vi "RT Driver VI.vi"(7 "Operation":T1, 11 "Device Reference in":T2 format="%.0x") -> (0 "Error Code":i32)   [LabVIEW 2017, in "Data Sharing Custom Device Engine.lvlib"]
uses:
  Data Sharing Custom Device Engine.lvlib
  <vilib>/NI Veristand/Custom Device API/Custom Device Item Ref.ctl
  <vilib>/NI Veristand/Custom Device API/Hardware Interface Driver VI Operation.ctl
  Builds/Data Sharing Framework/Current/Data Sharing Framework Core/Data Sharing Framework Core.lvlibp/Engine/Framework/Framework.lvclass
  Builds/Data Sharing Framework/Current/Data Sharing Framework Core/Data Sharing Framework Core.lvlibp/Engine/Internal/Configuration Classes/Framework Configuration/Framework Configuration.lvclass
  <vilib>/NI Veristand/Custom Device API/Custom Device API.lvlib
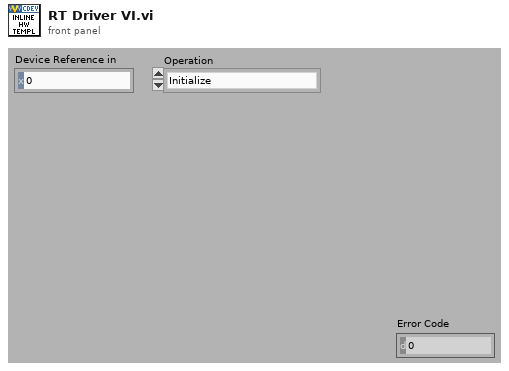
[diagram p1: front panel]
types:
  T1 = typedef "Custom Device API.lvlib/Hardware Interface Driver VI Operation.ctl" = enum16{"Initialize", "Start", "Read Data from HW", "Write Data to HW", "Close"}
  T2 = typedef "Custom Device API.lvlib/Custom Device Item Ref.ctl" = u64
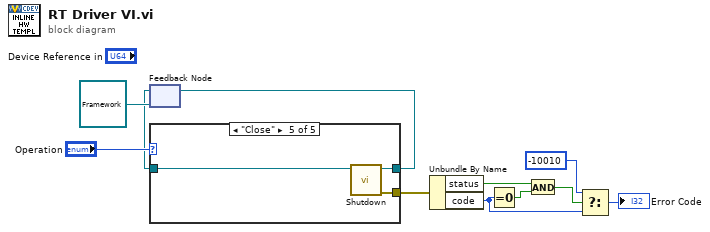
[diagram p0: block diagram]
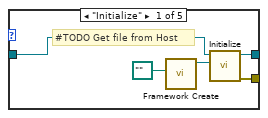
[diagram p2: hidden frame]
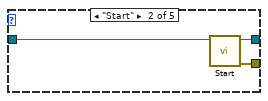
[diagram p3: hidden frame]
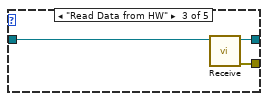
[diagram p4: hidden frame]
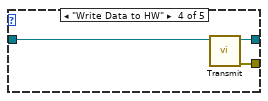
[diagram p5: hidden frame]
diagram:
  n1 = feedback #1(refnum<class "Framework.lvclass"> refnum ("Data Sharing Framework Core.lvlibp:Data Sharing Framework Engine.lvlib:Framework")) -> (w8:refnum<class "Framework.lvclass">)
  n2 = case shown="\"Close\"" "Operation" {
    tunnel: w8 -> [w16 w19 w22 w25 w26]
    tunnel: [w13 w18 w21 w24 w28] -> w9
    tunnel: [w12 w17 w20 w23 w27] -> w7
    frame "Initialize" {
      # "#TODO Get file from Host"
      n3 = call "Framework Create.vi"("configuration path"=path "") -> ("Framework Configuration"=w15:refnum<class "Framework Configuration.lvclass">)  [unwired: 9 in, 1 out]
      n4 = call "Initialize.vi"("Framework Configuration"=w15, "Framework type"=w16) -> ("error out"=w12:errorcluster, "Framework out"=w13:refnum<class "Framework.lvclass">)  [unwired: 8 in]
    }
    frame "Start" {
      n5 = call "Start.vi"("Framework in"=w19) -> ("error out"=w17:errorcluster, "Framework out"=w18:refnum<class "Framework.lvclass">)  [unwired: 9 in]
    }
    frame "Read Data from HW" {
      n6 = call "Receive.vi"("Framework in"=w22) -> ("error out"=w20:errorcluster, "Framework out"=w21:refnum<class "Framework.lvclass">)  [unwired: 9 in]
    }
    frame "Write Data to HW" {
      n7 = call "Transmit.vi"("Framework in"=w25) -> ("error out"=w23:errorcluster, "Framework out"=w24:refnum<class "Framework.lvclass">)  [unwired: 9 in]
    }
    frame "Close" {
      n8 = call "Shutdown.vi"("Framework in"=w26) -> ("error out"=w27:errorcluster, "Framework out"=w28:refnum<class "Framework.lvclass">)  [unwired: 9 in]
    }
  }
  n9 = feedback-in #1(w9) -> ()
  n10 = Unbundle By Name(w7) -> ("status"=w5:bool, "code"=w3:i32)
  n11 = Equal To 0?(x=w3) -> (x = 0?=w6:bool)
  n12 = And(x=w5, y=w6) -> (x .and. y?=w4:bool)
  n13 = Select(t=-10010, s=w4, f=w3) -> (s? t:f=→"Error Code":i32)
